vi "example 13 - child.vi"() -> ()   [LabVIEW 2020]
panel:
  in  "Multicolumn Listbox":i32(listbox)
  in  "Listbox":i32(listbox)
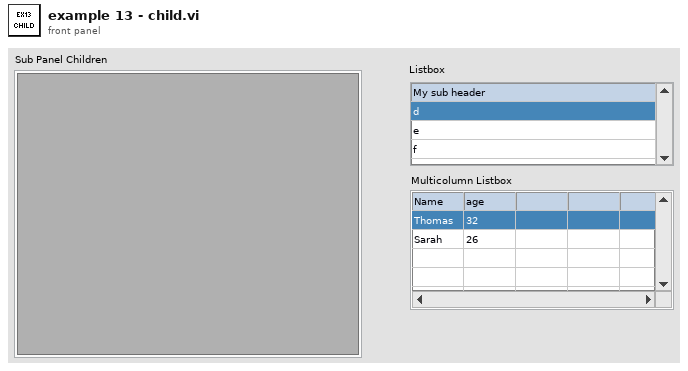
[diagram p1: front panel]
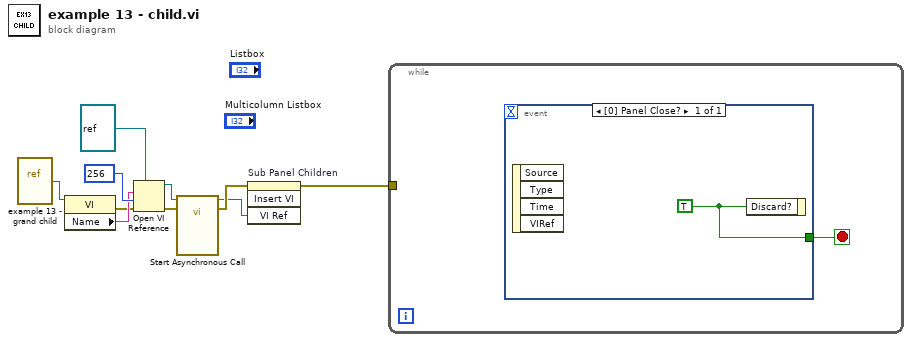
[diagram p0: block diagram]
diagram:
  n1 = vi-ref "example 13 - grand child.vi"() -> (w6:refnum<vi>)
  n2 = property class="VI"(reference=w6) -> (error out=w4:errorcluster, "Name"=w5:string)  [unwired: 1 in, 1 out]
  n3 = Open VI Reference(type specifier VI Refnum (for type only)=refnum<vi> refnum, vi path=w5, options=256 ("call and forget"), error in (no error)=w4) -> (vi reference=w8:refnum<vi>, error out=w7:errorcluster)  [unwired: 2 in]
  n4 = call-by-ref "Start Asynchronous Call"(reference=w8, error in=w7) -> (reference out=w2:refnum<vi>, error out=w3:errorcluster)  [unwired: 12 in]
  n5 = invoke on="Sub Panel Children" class="SubPnl" method="Insert VI"(error in=w3, "VI Ref"=w2) -> (error out=w1:errorcluster)  [unwired: 2 in, 3 out]
  n6 = while {
    tunnel: w1 -> [_]
    stop <- w11 stop-if-true
    n7 = event shown="[0] Panel Close?" {
      selector: _ -> [_]
      dyn-events: _ -> [_]
      timeout: _ -> [_]
      tunnel: [w12] -> w11
      event Panel Close? {
        w12 = TRUE
        n8 = event-data() -> ()  [unwired: 1 in, 4 out]
        n9 = event-data("Discard?"=w12) -> ()  [unwired: 1 in, 1 out]
      }
    }
  }
